vi "Test_Iso.vi"(8 "error in (no error)":errorcluster, 10 "Limits":T1, 11 "connection ID":refnum<k5>) -> (0 "error out":errorcluster, 2 "results":T2(array[cluster]), 3 "connection ID out":refnum<k5>)   [LabVIEW 2026]
panel:
  out "error out 2":errorcluster
  in  "error in (no error) 2":errorcluster
  out "connection ID out 2":refnum<k5>
  in  "connection ID 2":refnum<k5>
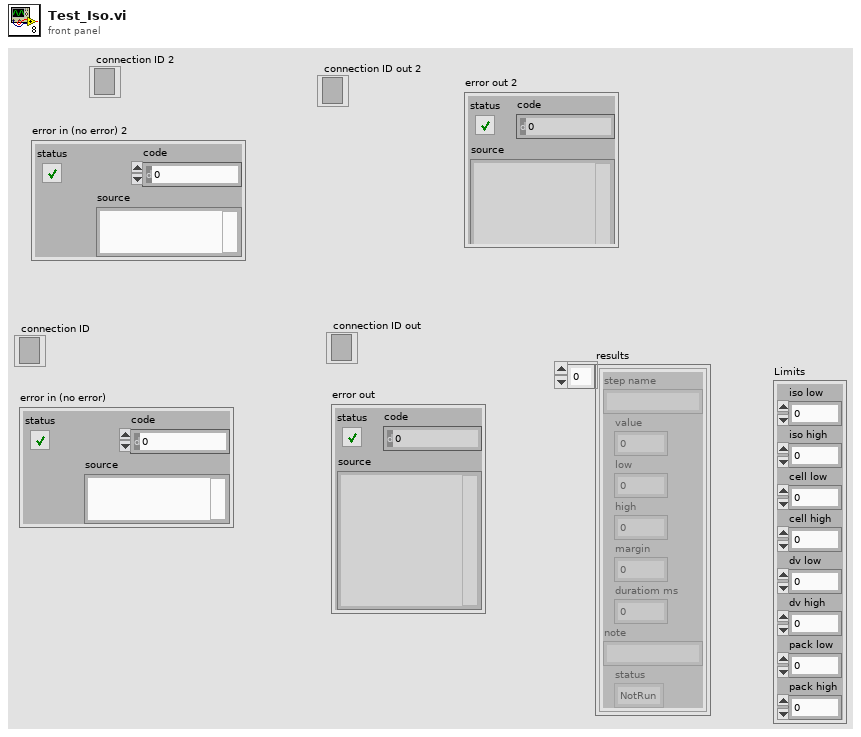
[diagram p1: front panel]
types:
  T1 = cluster{"iso low":dbl, "iso high":dbl, "cell low":dbl, "cell high":dbl, "dv low":dbl, "dv high":dbl, "pack low":dbl, "pack high":dbl}
  T2 = cluster{"step name":string, "value":dbl, "low":dbl, "high ":dbl, "margin":dbl, "duratiom ms":dbl, "note":string, "status":enum16{"NotRun", "Pass", "Fail", "Skipped"}}[]
  T3 = cluster{"step name":string, "value":dbl, "low":dbl, "high ":dbl, "margin":dbl, "duratiom ms":dbl, "note":string, "status":enum16{"NotRun", "Pass", "Fail", "Skipped"}}
  T4 = cluster{"step name":string, "value":dbl, "low":dbl, "high ":dbl, "margin":dbl, "duration ms":dbl, "note":string, "status":enum16{"NotRun", "Pass", "Fail", "Skipped"}}
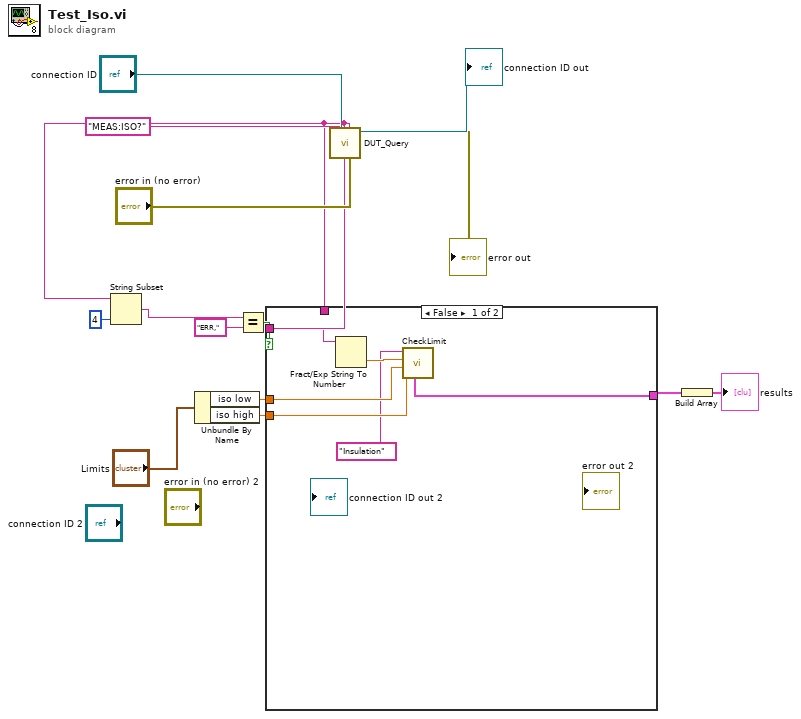
[diagram p0: block diagram]
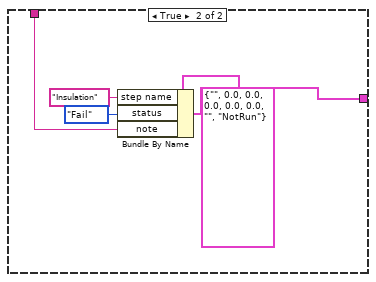
[diagram p2: hidden frame]
diagram:
  n1 = Unbundle By Name("Limits") -> ("iso low"=w5:dbl, "iso high"=w4:dbl)
  n2 = call "DUT_Query.vi"("error in (no error)"="error in (no error)", "command"="MEAS:ISO?", "connection ID"="connection ID") -> ("error out"=→"error out":errorcluster, "reply"=w3:string, "connection ID out"=→"connection ID out":refnum<k5>)  [unwired: 5 in, 1 out]
  n3 = String Subset(string=w3, length (rest)=4 ("length (rest)")) -> (substring=w9:string)  [unwired: 1 in]
  n4 = Equal?(x=w9, y="ERR,") -> (x = y?=w7:bool)
  n5 = case shown="False" w7 {
    tunnel: w3 -> [w21 _]
    tunnel: w5 -> [w19 _]
    tunnel: w4 -> [w18 _]
    tunnel: [w16 w22] -> w2
    tunnel: w3 -> [_ w23]
    frame False {
      n6 = Fract/Exp String To Number(string=w21) -> (number=w20:dbl)  [unwired: 3 in, 1 out]
      n7 = call "CheckLimit.vi"("high"=w18, "low"=w19, "value"=w20, "step name"="Insulation") -> ("Result"=w16:T4)  [unwired: 5 in, 2 out]
    }
    frame True {
      n8 = Bundle By Name(cluster=T3 {"step name"="", "value"=0.0, "low"=0.0, "high "=0.0, "margin"=0.0, "duratiom ms"=0.0, "note"="", "status"=enum."NotRun"} ("Result"), "step name"="Insulation", "status"=enum16{"NotRun", "Pass", "Fail", "Skipped"}."Fail", "note"=w23) -> (w22:T3)
    }
  }
  n9 = Build Array(w2) -> (→"results":T2)
